vi "LVClass_ComputePhaseSet GetZonalFilter.vi"(0 "ComputePhaseSet in":refnum<class "ComputePhaseSet.lvclass">, 11 "error in (no error)":errorcluster) -> (4 "ComputePhaseSet out":refnum<class "ComputePhaseSet.lvclass">, 6 "numero_zonal_to_filter":u8[](array[numeric]), 15 "error out":errorcluster)   [LabVIEW 2020, in "ComputePhaseSet.lvclass"]
doc: "Get filter for zonal phase reconstruction. The filter is defined by the\nindices of array params that must be filtered. see\nImop_ComputePhaseSet_GetLegendreFilter for details.\n\n--------------------------------------------------------------------------------\n\n<B>ComputePhaseSetIn </B> : ComputePhaseSet object.\n<B>ComputePhaseSetOut </B> : ComputePhaseSet object.\n<B>params </B> : Array of aberrations to filter.\n<B>ErrorIn </B> : Error\n<B>ErrorOut </B> : Error\n\n--------------------------------------------------------------------------------"
uses:
  ComputePhaseSet.lvclass
  ComputePhaseSet.lvclass/ComputePhaseSet.ctl
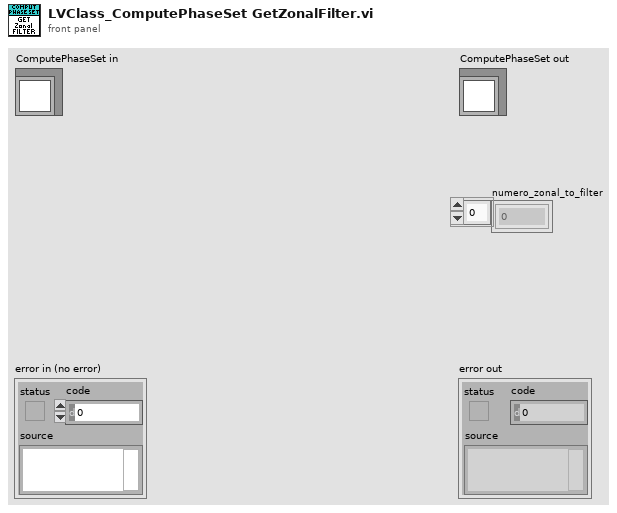
[diagram p1: front panel]
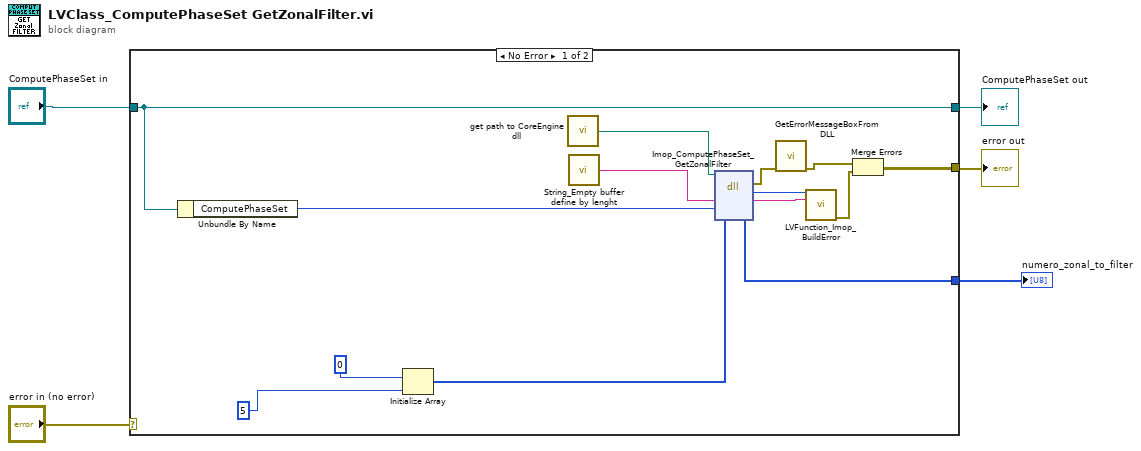
[diagram p0: block diagram]
diagram:
  n1 = case shown="No Error" "error in (no error)" {
    selector: "error in (no error)" -> [_ w21]
    tunnel: [w9 w21] -> w2
    tunnel: [w13 w20] -> w4
    tunnel: "ComputePhaseSet in" -> [w13 w20]
    tunnel: [w6 _] -> w1
    frame No Error {
      n2 = Unbundle By Name(w13) -> ("ComputePhaseSet"=w14:i32)
      n3 = Initialize Array(u8 0, 5 ("y")) -> (w7:u8[])
      n4 = call "get path to CoreEngine dll.vi"() -> ("path to c_interface_vc100.dll"=w16:path)  [unwired: 12 in, 3 out]
      n5 = call "String_Empty buffer define by lenght.vi"() -> ("Empty buffer"=w17:string)  [unwired: 1 in]
      n6 = dll-call lib="D:/2_trunk/Soft_haso/ImOpCoreEngine4_LV2011/DLLs/ImopEngine4_vc100.dll" fn="Imop_ComputePhaseSet_GetZonalFilter"(path in=w16, "message"=w17, "objet"=w14, "param"=w7) -> (error out=w15:errorcluster, "return type"=w19:i32, "message"=w18:string, "param"=w6:u8[])  [unwired: 3 in, 1 out]
      n7 = call "GetErrorMessageBoxFromDLL.vi"("error IN"=w15) -> ("error OUT"=w11:errorcluster)  [unwired: 10 in]
      n8 = call "LVFunction_Imop_BuildError.vi"("code"=w19, "String to Prepend to source (\"\")"=w18) -> ("error out"=w10:errorcluster)  [unwired: 13 in]
      n9 = Merge Errors(w11, w10) -> (w9:errorcluster)
    }
    frame Error {
    }
  }
  "error out" <- w2
  "ComputePhaseSet out" <- w4
  "numero_zonal_to_filter" <- w1
